vi "Generate Unique Header.vi"(8 "error in (no error)":errorcluster, 11 "ePAS Data in":refnum<class "ePAS Data.lvclass">) -> (0 "error out":errorcluster, 2 "Header":string[](array[string]), 3 "ePAS Data out":refnum<class "ePAS Data.lvclass">)   [LabVIEW 2014, in "ePAS Library.lvlib" / "ePAS Data.lvclass"]
uses:
  ePAS Data.lvclass
  reusable/Data/Data.lvlibp/Read Data ID.vi
  reusable/PAS/Data/Main/PAS Data.lvclass
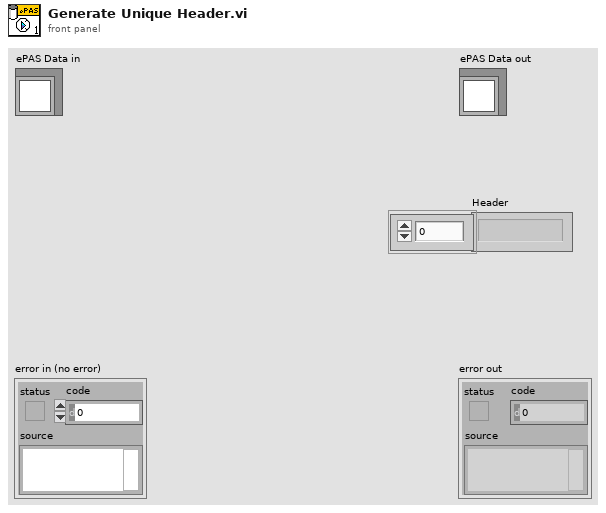
[diagram p1: front panel]
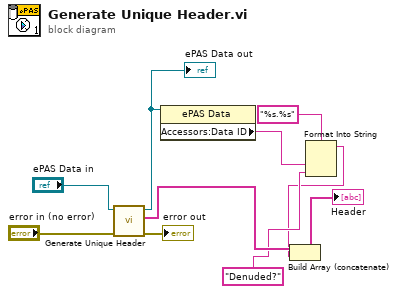
[diagram p0: block diagram]
diagram:
  n1 = call-parent "Generate Unique Header.vi"("error in (no error)"="error in (no error)", "PAS Data in"="ePAS Data in") -> ("error out"=→"error out":errorcluster, "Header"=w7:string[], "PAS Data out"=w5:refnum<class "ePAS Data.lvclass">)  [unwired: 7 in]
  "ePAS Data out" <- w5
  n2 = property class="ePAS Data"(reference=w5) -> ("Accessors:Data ID"=w3:string)  [unwired: 1 in, 2 out]
  n3 = Format Into String(format string="%s.%s", w3, "Denuded?") -> (resulting string=w1:string)  [unwired: 2 in, 1 out]
  n4 = Build Array (concatenate)(w7, w1) -> (→"Header":string[])
